vi "Main.vi"(11 "Module Admin":refnum<class "Delacor_lib_QMH_Module Admin.lvclass">) -> ()   [LabVIEW 2019, in "Panther Dashboard.lvlib"]
doc: "Panther Dashboard For DQMH®\n\nDeveloped and maintained by:\nPantherLAB\n\nMain Contributor- Developer:\n\n» Enrique Noé Arias\n\nBrainstorming & Code Reviews:\n\n» Matthias Baudot\n» Fabiola De La Cueva\n» Christopher Farmer\n» Cyril Gambini\n» Joerg Hampel\n» Olivier Jourdan\n» Cesar Muñoz\n» Darren Nattinger\n» Luis Orozco\n» Sam Taggart\n» Diego Torres"
uses:
  Panther Dashboard.lvlib
  <vilib>/Delacor/Delacor QMH/Libraries/Module Admin_class/Delacor_lib_QMH_Module Admin.lvclass
  Module Data--cluster.ctl
  Maps List and refs--cluster.ctl
  <vilib>/National Instruments/Tree Map/Tree Map Data.ctl
  DQMH Modules Info--cluster.ctl
  Module type--enum.ctl
  Project References--cluster.ctl
  Selection Type--enum.ctl
  References Updated Argument--cluster.ctl
  Launch DQMH Scripting Tools Argument--cluster.ctl
  DQMH Tools Menu--enum.ctl
  <vilib>/Delacor/Delacor QMH/Libraries/Message Queue_class/Delacor_lib_QMH_Message Queue.lvclass/Delacor_lib_QMH_Message Queue.ctl
  Expand Results Argument--cluster.ctl
  Execute Default Event Request Argument--cluster.ctl
  Tree DQMH Selection Argument--cluster.ctl
  Scan DQMH Modules Argument--cluster.ctl
  Stop Argument--cluster.ctl
  Generate Project Documentation Argument--cluster.ctl
  Set App Theme Argument--cluster.ctl
  Show About Argument--cluster.ctl
  Update Module ID Argument--cluster.ctl
  Save Library Description Argument--cluster.ctl
  Save VI Description Argument--cluster.ctl
  Open Documentation Argument--cluster.ctl
  Save Project Documentation Argument--cluster.ctl
  <vilib>/Delacor/Delacor QMH/Libraries/Module Admin_class/Delacor_lib_QMH_Module Admin.lvclass/Delacor_lib_QMH_Module Admin.ctl
  <vilib>/Delacor/Delacor QMH/Libraries/Message Queue_class/Delacor_lib_QMH_Enqueue Message (Single).vi
  <vilib>/Delacor/Delacor QMH/Libraries/Module Admin_class/Delacor_lib_QMH_Get External Launch.vi
  Panther Dashboard--global.vi
  <vilib>/National Instruments/Tree Map/API/List Roots.vi
  <vilib>/National Instruments/Tree Map/Utility/Into Tree Control Items.vi
  <vilib>/Platform/browser.llb/Open URL in Default Browser (path).vi
  <vilib>/Utility/error.llb/Error Cluster From Error Code.vi
  <vilib>/ErrorRing/Error Ring.xnode
  <vilib>/Delacor/Delacor QMH/Libraries/Message Queue_class/Delacor_lib_QMH_Message Queue.lvclass
  <vilib>/National Instruments/Tree Map/Tree Map.lvlib
  <vilib>/Delacor/Delacor QMH/Libraries/Scripting API/DQMH_Scripting API.lvlib
  ContextHelp/ContextHelp.lvlib
panel:
  out "error out":errorcluster
  in  "Context Help Panther":bool caption="Doc Editor"
  in  "Add Event":bool
  in  "Remove Event":bool caption="Remove"
  in  "Convert Event":bool caption="Convert"
  in  "Rename Event":bool caption="Rename"
  in  "Add New Module":bool caption="Add"
  in  "Rename Module":bool caption="Rename"
  in  "Validate Module":bool caption="Validate"
  in  "Create Module Template":bool caption="Template"
  in  "Add Unit Test Module":bool caption="Unit Test"
  in  "Create RT Tester Module":bool caption="RT Tester"
  in  "Open Antidoc Output":bool caption="Open"
  in  "Generate Antidoc":bool caption="Antidoc"
  in  "About Panther":bool caption="About"
  in  "Theme Panther":bool caption="Theme"
  in  "Projects":string(combo)
  in  "Targets":string(combo)
  in  "Search":bool caption="Scan Project"
  in  "Expand Results":bool
  in  "Include Dependencies":bool
  in  "Module ID":i32=-1 min=-1 max=1000 step=1 format="Module ID %d"
  in  "Modules Tree":string(tree) caption="Tree 2"
  out "antidoc":bool
  out "Panther Indicator":bool
  out "Process Indicator":bool
  out "Event Indicator":bool
  out "Status":string
  out "Progress":u16(slide) scale=-1.0..4.0
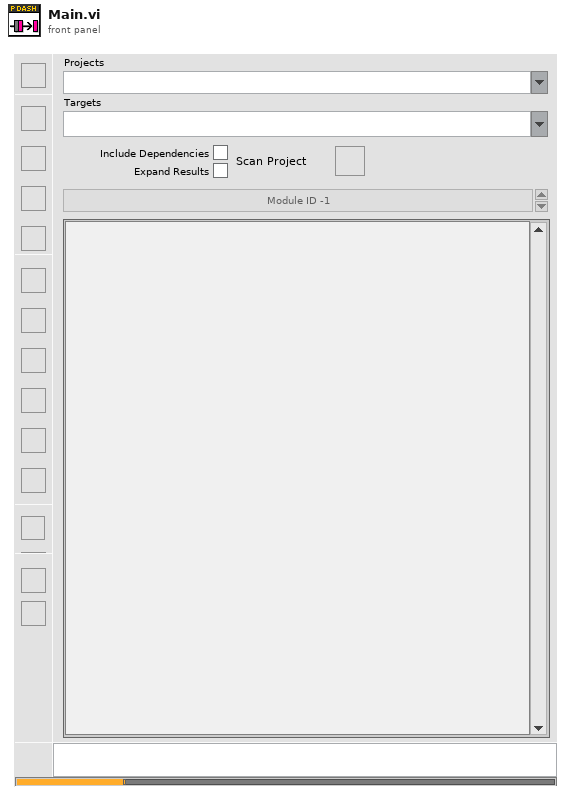
[diagram p1: front panel]
types:
  T1 = typedef "Panther Dashboard.lvlib/Broadcast Events--cluster.ctl" = cluster{"Module Did Init":refnum<user-event>, "Status Updated":refnum<user-event>, "Error Reported":refnum<user-event>, "Module Did Stop":refnum<user-event>, "Update Module Execution Status":refnum<user-event>, "References Updated":refnum<user-event>, "Projects Updated":refnum<user-event>, "Targets Updated":refnum<user-event>, "Progress updated":refnum<user-event>, "Scale Updated":refnum<user-event>, "Connector Pane Updated":refnum<user-event>, "Documentation Updated":refnum<user-event>, "Module Type Updated":refnum<user-event>, "Theme Updated":refnum<user-event>, "Project Description Updated":refnum<user-event>}
  T2 = typedef "Panther Dashboard.lvlib/Request Events--cluster.ctl" = cluster{"Stop Module":refnum<user-event>, "Show Panel":refnum<user-event>, "Hide Panel":refnum<user-event>, "Get Module Execution Status":refnum<user-event>, "Show Diagram":refnum<user-event>, "Scan DQMH Modules":refnum<user-event>, "Tree DQMH Selection":refnum<user-event>, "Open Module API Tester":refnum<user-event>, "Execute Default Event Request":refnum<user-event>, "Expand Results":refnum<user-event>, "Launch DQMH Scripting Tools":refnum<user-event>, "Generate Project Documentation":refnum<user-event>, "Set App Theme":refnum<user-event>, "Show About":refnum<user-event>, "Update Module ID":refnum<user-event>, "Save Library Description":refnum<user-event>, "Save VI Description":refnum<user-event>, "Open Documentation":refnum<user-event>, "Save Project Documentation":refnum<user-event>, "Register controls Mouse Enter":refnum<user-event>}
  T3 = typedef "ContextHelp.lvlib/Broadcast Events--cluster.ctl" = cluster{"Module Did Init":refnum<user-event>, "Status Updated":refnum<user-event>, "Error Reported":refnum<user-event>, "Module Did Stop":refnum<user-event>, "Update Module Execution Status":refnum<user-event>}
  T4 = typedef "Panther Dashboard.lvlib/Selection Type--enum.ctl" = enum16{"Broadcast", "Request", "Module", "Public API"}
  T5 = typedef "Panther Dashboard.lvlib/Module Data--cluster.ctl" = cluster{"Maps":T6, "DQMH Scan Results":T8, "Current Selection":cluster{"VI Ref":refnum<vi>, "DQMH Lib Ref":refnum<vi>}, "Module type":T9, "Module ID":i32, "Theme":bool, "Broadcast?":bool}
  T6 = typedef "Panther Dashboard.lvlib/Maps List and refs--cluster.ctl" = cluster{"Tree Map":T7, "References Map":map{string, refnum<vi>}}
  T7 = typedef "Tree Map.lvlib/Tree Map Data.ctl" = map{string, cluster{"Child Paths Set":set{string}, "Name":string, "Data":string, "Attributes":map{string, string}}}
  T8 = typedef "Panther Dashboard.lvlib/DQMH Modules Info--cluster.ctl" = cluster{"All DQMH Modules Refs":refnum<vi>[], "All Modules Descriptions":string[], "All Modules type":T9[], "Project References":T10}
  T9 = typedef "Panther Dashboard.lvlib/Module type--enum.ctl" = enum16{"Module type: Singleton", "Module type: Cloneable"}
  T10 = typedef "Panther Dashboard.lvlib/Project References--cluster.ctl" = cluster{"Project Ref":refnum<vi>, "Project Name":string, "Target":refnum<vi>, "App Ref":refnum<vi>}
  T11 = typedef "Panther Dashboard.lvlib/References Updated Argument--cluster.ctl" = cluster{"Modules":refnum<vi>[], "Modules Types":T9[], "Application Instance":refnum<vi>}
  T12 = enum8{"Enabled", "Disabled", "Disabled and Grayed Out"}
  T13 = typedef "Panther Dashboard.lvlib/Launch DQMH Scripting Tools Argument--cluster.ctl" = cluster{"Scripting Tool":T14}
  T14 = typedef "Panther Dashboard.lvlib/DQMH Tools Menu--enum.ctl" = enum16{"Create New DQMH Event", "Remove DQMH Event", "Convert DQMH Event", "Rename DQMH Event", "Add New DQMH Module", "Create RT Tester", "Rename DQMH Module", "Validate DQMH Module", "Create DQMH Module Template", "New DQMH  Unit Test"}
  T15 = typedef "Panther Dashboard.lvlib/Expand Results Argument--cluster.ctl" = cluster{"Expand?":bool}
  T16 = typedef "Panther Dashboard.lvlib/Execute Default Event Request Argument--cluster.ctl" = cluster{"Event Name":string}
  T17 = typedef "Panther Dashboard.lvlib/Tree DQMH Selection Argument--cluster.ctl" = cluster{"Tree DQMH Sel":string}
  T18 = typedef "Panther Dashboard.lvlib/Scan DQMH Modules Argument--cluster.ctl" = cluster{"Include Dependencies":bool, "Project":string, "Target":string}
  T19 = enum32{"invalid lock state", "Not Locked", "Locked (No Password)", "Password-protected"}
  T20 = typedef "Panther Dashboard.lvlib/Stop Argument--cluster.ctl" = cluster{"Origin":string, "Exit via Stop Module Req?":bool, "Wait for Module to stop?":bool}
  T21 = typedef "Panther Dashboard.lvlib/Generate Project Documentation Argument--cluster.ctl" = cluster{"Boolean":bool}
  T22 = typedef "Panther Dashboard.lvlib/Set App Theme Argument--cluster.ctl" = cluster{"Theme":bool}
  T23 = typedef "Panther Dashboard.lvlib/Show About Argument--cluster.ctl" = cluster{"Boolean":bool}
  T24 = typedef "Panther Dashboard.lvlib/Update Module ID Argument--cluster.ctl" = cluster{"New ID":i32}
  T25 = typedef "Panther Dashboard.lvlib/Save Library Description Argument--cluster.ctl" = cluster{"Library Description":string}
  T26 = typedef "Panther Dashboard.lvlib/Save VI Description Argument--cluster.ctl" = cluster{"VI Description":string}
  T27 = typedef "Panther Dashboard.lvlib/Open Documentation Argument--cluster.ctl" = cluster{"Boolean":bool}
  T28 = typedef "Panther Dashboard.lvlib/Save Project Documentation Argument--cluster.ctl" = cluster{"Project Description":string}
  T29 = cluster{"Left Cell String":string, "Child Text":string[], "Child Tag":string, "Item Indent":i32, "Child Only?":bool, "Glyph Index":i32}[]
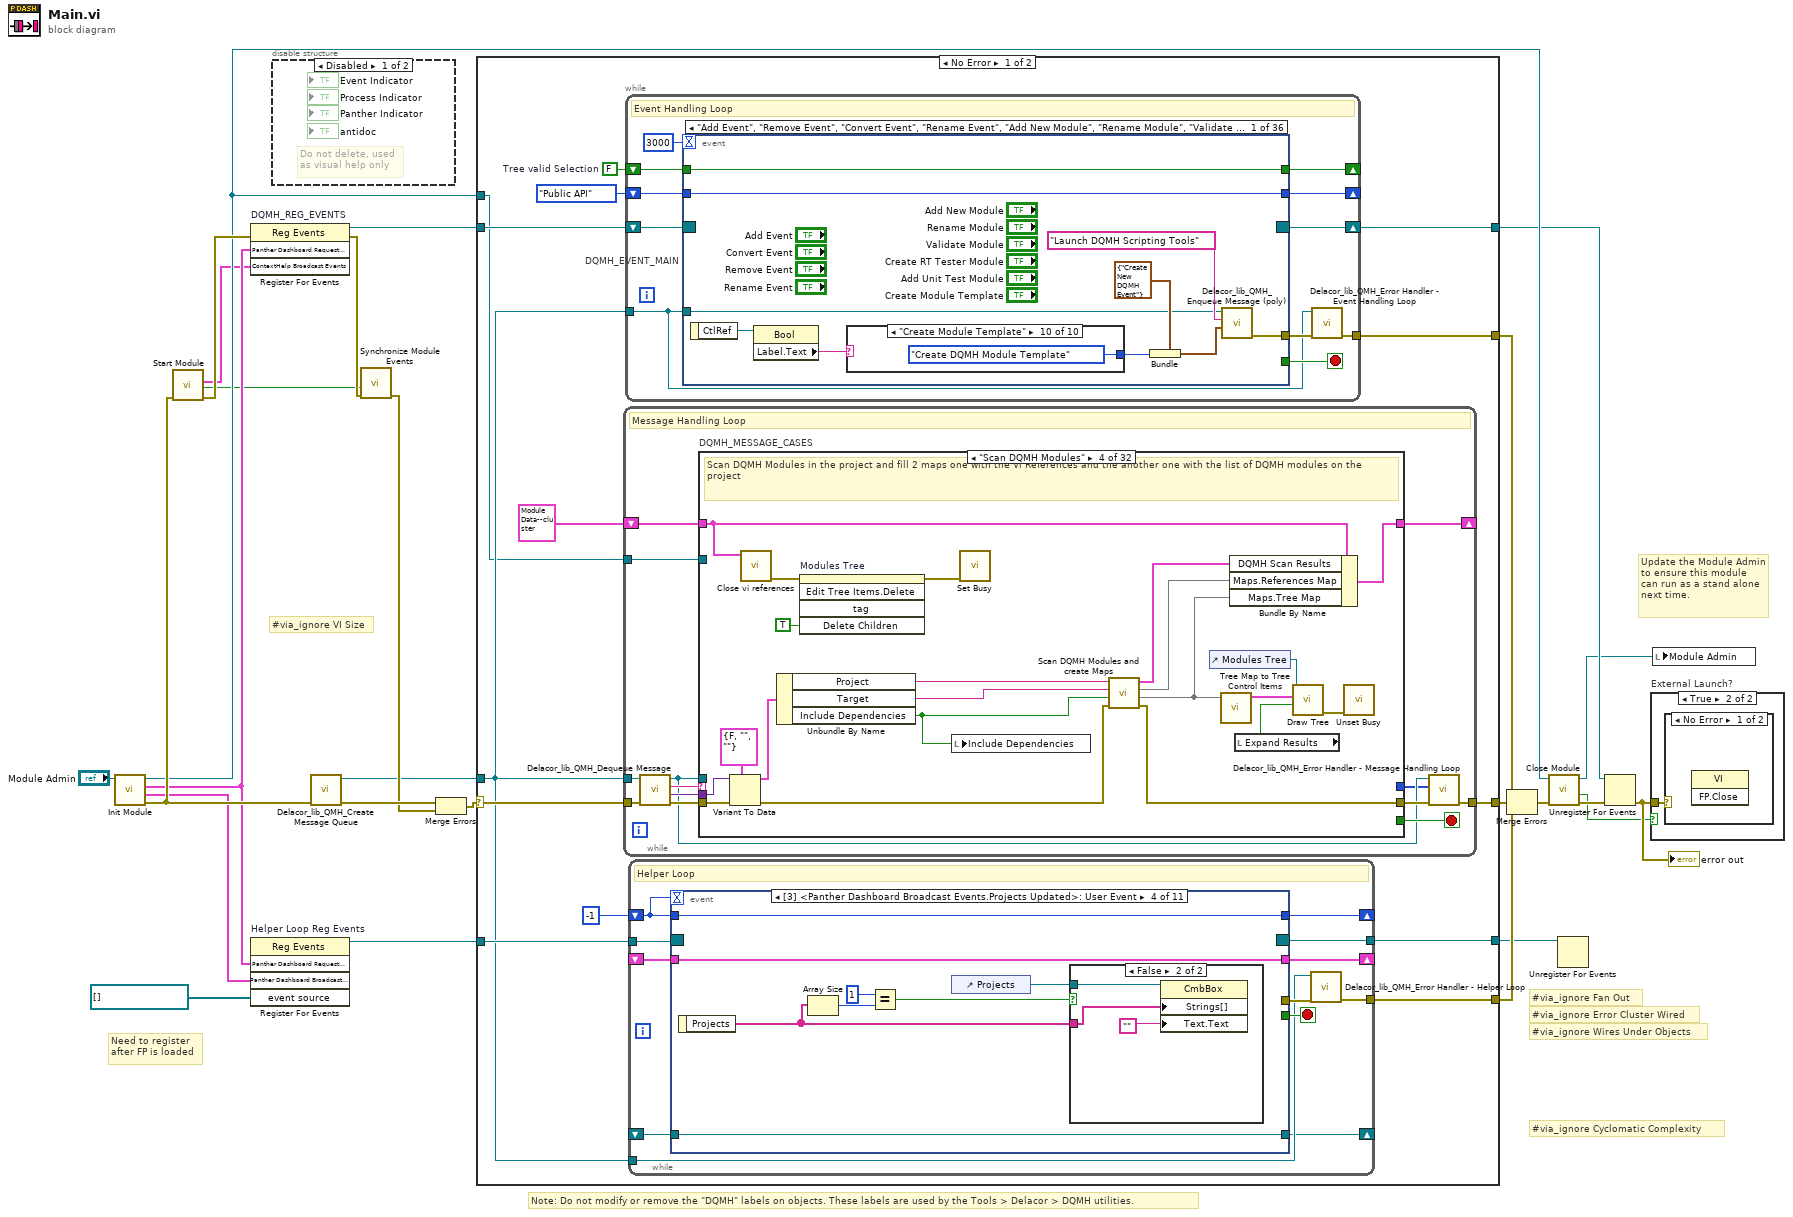
[diagram p0: block diagram]
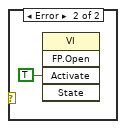
[diagram p4: hidden frame]
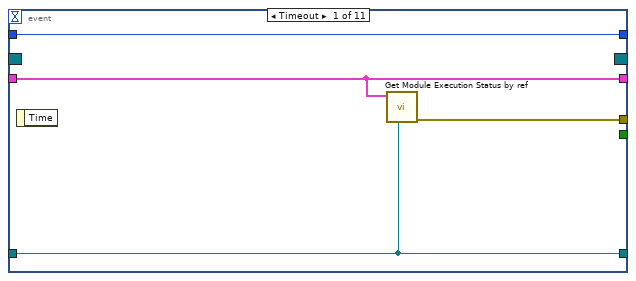
[diagram p5: hidden frame]
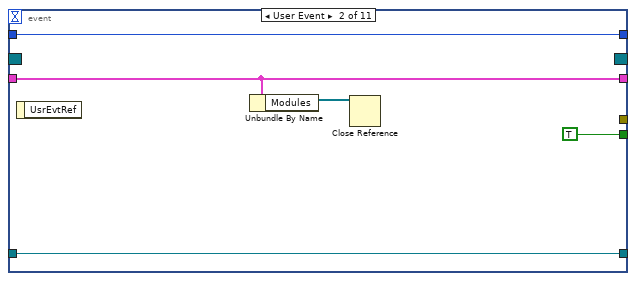
[diagram p6: hidden frame]
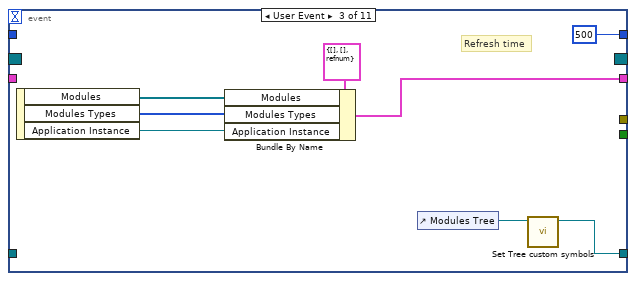
[diagram p7: hidden frame]
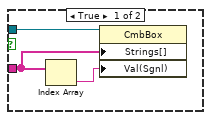
[diagram p8: hidden frame]
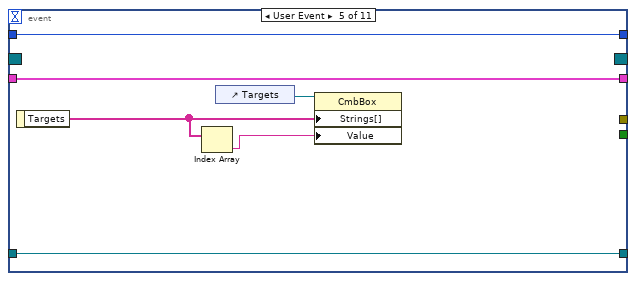
[diagram p9: hidden frame]
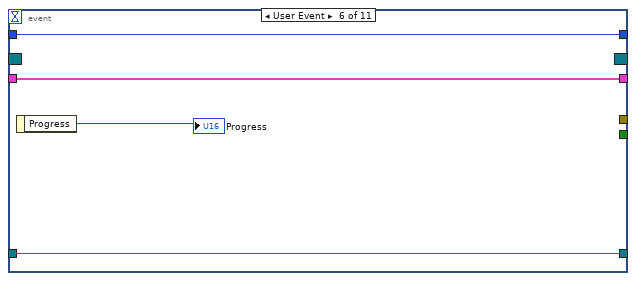
[diagram p10: hidden frame]
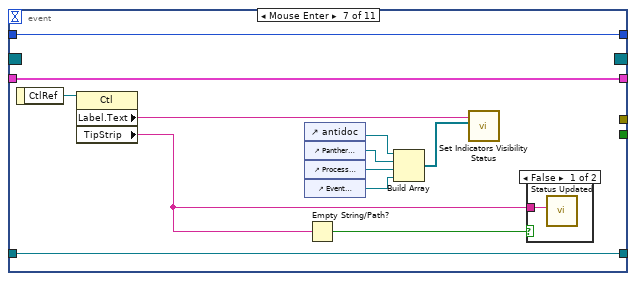
[diagram p11: hidden frame]
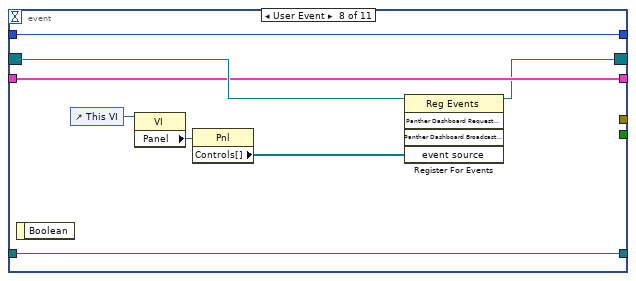
[diagram p13: hidden frame]
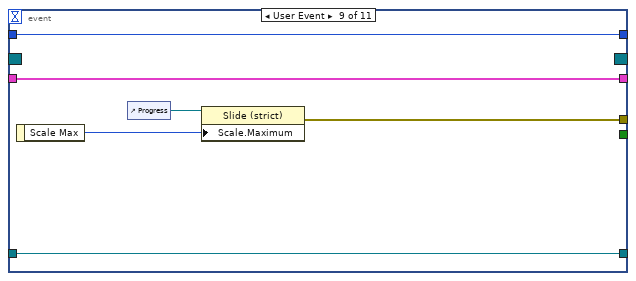
[diagram p14: hidden frame]
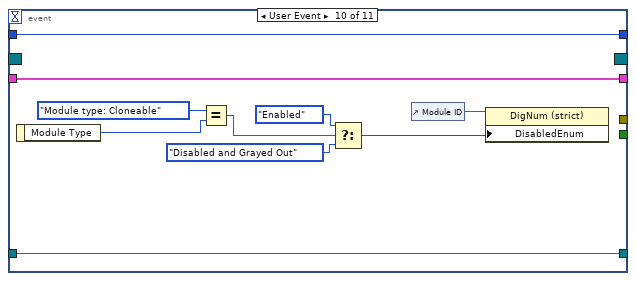
[diagram p15: hidden frame]
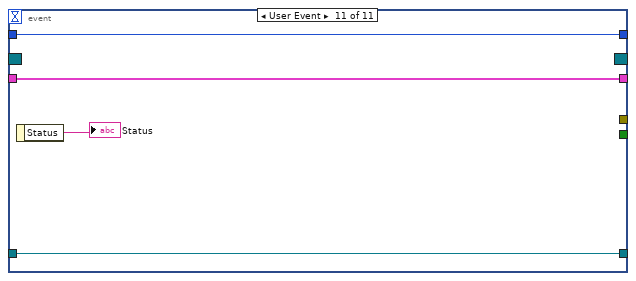
[diagram p16: hidden frame]
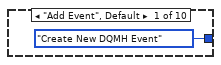
[diagram p17: hidden frame]
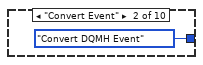
[diagram p18: hidden frame]
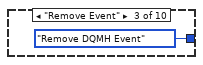
[diagram p19: hidden frame]
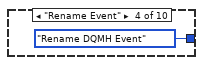
[diagram p20: hidden frame]
diagram:
  # "Need to register\nafter FP is loaded"
  # "#via_ignore VI Size"
  # "#via_ignore Fan Out"
  # "#via_ignore Cyclomatic Complexity"
  # "#via_ignore Wires Under Objects"
  # "#via_ignore Error Cluster Wired"
  # "Note: Do not modify or remove the \"DQMH\" labels on objects. These labels are used by the Tools > Delacor > DQMH utilities."
  # "Update the Module Admin to ensure this module can run as a stand alone next time."
  n1 = call "Init Module.vi"("Singleton Module Admin in"="Module Admin") -> ("error out"=w15:errorcluster, "Panther Dashboard Broadcast Events"=w4:T1, "Panther Dashboard Request Events"=w5:T2, "Singleton Module Admin out"=w14:refnum<class "Delacor_lib_QMH_Module Admin.lvclass">)  [unwired: 7 in]
  n2 = call "Start Module.vi"("error in"=w15) -> ("error out"=w17:errorcluster, "Wait for Event Sync?"=w3:bool, "ContextHelp Broadcast Events"=w2:T3)  [unwired: 7 in, 1 out]
  n3 = register-events "DQMH_REG_EVENTS"(error in=w17, w5, w2) -> (reference out=w12:refnum<event-registration>, error out=w18:errorcluster)  [unwired: 1 in]
  n4 = register-events "Helper Loop Reg Events"(w5, w4, refnum<vi>[] [] ("event source")) -> (reference out=w7:refnum<event-registration>)  [unwired: 2 in, 1 out]
  n5 = disable-structure shown="Disabled" {
    frame Disabled {
      # "Do not delete, used\nas visual help only"
    }
    frame Enabled {
    }
  }
  n6 = call <vilib>:"Delacor_lib_QMH_Create Message Queue.vi"("error in"=w15) -> ("error out"=w21:errorcluster, "Message Queue"=w11:refnum<class "Delacor_lib_QMH_Message Queue.lvclass">)  [unwired: 9 in]
  n7 = call "Synchronize Module Events.vi"("error in"=w18, "Wait for Event Sync?"=w3) -> ("error out"=w16:errorcluster)  [unwired: 9 in]
  n8 = Merge Errors(w21, w16) -> (w20:errorcluster)
  n9 = case shown="No Error" w20 {
    selector: w20 -> [w38 w805]
    tunnel: [w40 w804] -> w26
    tunnel: [w36 w803] -> w13
    tunnel: w12 -> [w34 w803]
    tunnel: w11 -> [w30 w799]
    tunnel: [w39 _] -> w24
    tunnel: w14 -> [w27 w800]
    tunnel: w7 -> [w33 w798]
    tunnel: [w32 w798] -> w6
    tunnel: [w37 _] -> w19
    frame No Error {
      w29 = FALSE  # Tree valid Selection
      n10 = while {
        tunnel: w30 -> [w451]
        shift-right: [w455] -> _
        shift-left: T5 {"Maps"={"Tree Map"={}, "References Map"={}}, "DQMH Scan Results"={"All DQMH Modules Refs"=[], "All Modules Descriptions"=[], "All Modules type"=[], "Project References"={"Project Ref"=refnum, "Project Name"="", "Target"=refnum, "App Ref"=refnum}}, "Current Selection"={"VI Ref"=refnum, "DQMH Lib Ref"=refnum}, "Module type"=enum."Module type: Singleton", "Module ID"=0, "Theme"=FALSE, "Broadcast?"=FALSE} ("Data Cluster") -> [w456]
        tunnel: w38 -> [w459]
        tunnel: [w457] -> w40
        tunnel: w27 -> [w449]
        stop <- w454 stop-if-true
        # "Message Handling Loop"
        n11 = call-dynamic "Delacor_lib_QMH_Dequeue Message.vi"("error in"=w459, "Message Queue in"=w451) -> ("error out"=w458:errorcluster, "Message Data"=w452:variant, "Message"=w453:string, "Message Queue out"=w450:refnum<class "Delacor_lib_QMH_Message Queue.lvclass">)  [unwired: 6 in]
        n12 = case "DQMH_MESSAGE_CASES" shown="\"Scan DQMH Modules\"" w453 {
          selector: w453 -> [_ w484 _ _ _ _ _ _ _ _ _ _ _ _ _ _ _ _ _ _ _ _ _ _ _ _ _ _ _ _ _ w784]
          tunnel: w450 -> [_ _ _ _ _ _ _ _ _ _ _ _ _ _ _ _ _ _ _ _ _ _ _ _ _ _ _ _ _ w753 w776 _]
          tunnel: w458 -> [w481 w489 w491 w512 w519 w526 w533 w548 w557 w562 w568 w582 w595 w617 w623 w630 w637 w642 w655 w664 w675 w684 w692 w702 w718 w734 w745 w748 w750 w760 w782 w786]
          tunnel: [w475 w487 w491 w511 w518 w526 w533 w547 w556 w563 w569 w580 w593 w618 w622 w629 w636 w641 w653 w662 w672 w680 w691 w700 w716 w733 w743 w747 w750 w756 w779 w787] -> w460
          tunnel: w456 -> [w472 w486 w490 w498 w516 w524 w532 w543 w555 w561 w567 w575 w592 w616 w621 w628 w635 w640 w644 w658 w671 w679 w690 w694 w711 w723 w739 w746 w749 w755 w768 w785]
          tunnel: [w471 w486 w490 w503 w516 w524 w532 w539 w555 w561 w567 w575 w592 w616 w621 w626 w635 w640 w644 w658 w666 w679 w686 w693 w709 w723 w739 w746 w749 w755 w768 w785] -> w455
          tunnel: [_ _ _ _ _ _ _ _ _ _ _ _ _ _ _ _ _ _ _ _ _ _ _ _ _ _ _ _ _ _ w775 _] -> w454
          tunnel: w452 -> [_ w485 _ w506 _ _ _ w546 _ _ _ w578 _ _ _ w627 w634 _ w652 w660 w670 w678 w689 w698 w714 w732 w742 _ _ w754 w774 _]
          tunnel: w449 -> [w473 _ _ _ _ _ _ _ _ _ _ _ _ _ _ _ _ _ _ _ _ _ _ _ _ _ _ _ _ w752 w769 _]
          tunnel: [_ _ _ _ _ _ _ _ _ _ _ _ i32[] [5000, 1026, 43] ("specific error code to clear (0: all)") _ _ _ _ _ _ _ _ _ _ _ _ _ _ _ _ _ _ _] -> w448
          frame "Initialize" {
            w462 = "Panther Dashboard for DQMH" ("format string")
            # "Initialize - Any operation that needs to be done before the module can receive messages. Synchronize Caller Events.vi will inform Start Module.vi that the module has launched and is ready to receive messages. Module Did Init.vi will broadcast that the module initialized."
            n13 = call "Synchronize Caller Events.vi"("error in (no error)"=w481, "Singleton Module Admin in"=w473) -> ("error out"=w480:errorcluster)  [unwired: 8 in, 1 out]
            n14 = property on="Modules Tree" class="Tree (strict)"("Allow Item Drag"=TRUE ("Drag/Drop:Allow Dragging"), "SelColor"=u32 8355711) -> ()  [unwired: 2 in, 2 out]
            n15 = call "Module Name--constant.vi"() -> ("Module Name"=w469:string)  [unwired: 11 in]
            n16 = call "Module Did Init.vi"("error in (no error)"=w480, "Initialized?"=TRUE, "Origin"=w469) -> ("error out"=w479:errorcluster)  [unwired: 8 in]
            n17 = control-ref of="Projects"() -> (w465:refnum<vi>)
            n18 = call "Scan For App Projects.vi"("error in"=w479, "Init?"=TRUE, "Projects Ref"=w465) -> ("error out"=w478:errorcluster)  [unwired: 8 in]
            n19 = call "Read Theme from Config.vi"("error in"=w478) -> ("error out"=w477:errorcluster, "Theme"=w461:bool)  [unwired: 9 in]
            n20 = local write "Theme Panther"(w461) -> ()
            n21 = call "Set App Theme.vi"("error in"=w477, "Theme"=w461) -> ("error out"=w476:errorcluster)  [unwired: 9 in]
            n22 = control-ref of="This VI"() -> (w463:refnum<vi>)
            n23 = Bundle By Name(cluster=w472, "Module ID"=-1) -> (w471:T5)
            n24 = call "Status Updated.vi"("Status"=w462) -> ()  [unwired: 10 in, 1 out]
            n25 = call "Set Panel Initial State.vi"("Title"=w462, "Main Vi Ref"=w463) -> ("error out"=w474:errorcluster)  [unwired: 9 in]
            n26 = Merge Errors(w474, w476) -> (w475:errorcluster)
          }
          frame "Refresh Targets" {
            # "When the User selects a Project triggers this task to scan all the targets available"
            n27 = Variant To Data(error in=w489, type=w484, Variant=w485) -> (data=w483:string, error out=w488:errorcluster)
            n28 = call "Get all Targets.vi"("error in"=w488, "Project Selection"=w483) -> ("error out"=w487:errorcluster, "Targets"=w482:string[])  [unwired: 8 in]
            n29 = call "Targets Updated.vi"("Targets"=w482) -> ()  [unwired: 10 in, 1 out]
          }
          frame "---Module Specific---" {
            # "Separator -- The following cases handle messages specific to this Module."
          }
          frame "Scan DQMH Modules" {
            # "Scan DQMH Modules in the project and fill 2 maps one with the Vi References and the another one with the list of DQMH modules on the project"
            n30 = Variant To Data(error in=w512, type=T18 {"Include Dependencies"=FALSE, "Project"="", "Target"=""} ("Scan DQMH Modules Argument"), Variant=w506) -> (data=w504:T18, error out=w509:errorcluster)
            n31 = call "Close vi references.vi"("Data Cluster"=w498) -> ("error out"=w508:errorcluster)  [unwired: 10 in]
            n32 = Unbundle By Name(w504) -> ("Project"=w494:string, "Target"=w496:string, "Include Dependencies"=w497:bool)
            n33 = invoke on="Modules Tree" class="Tree (strict)" method="Edit Tree Items.Delete"(error in=w508, "Delete Children"=TRUE ("Delete Children?")) -> (error out=w507:errorcluster)  [unwired: 3 in, 4 out]
            n34 = local write "Include Dependencies"(w497) -> ()
            n35 = call <vilib>:"Set Busy.vi"("error in (no error)"=w507) -> ()  [unwired: 9 in, 2 out]
            n36 = call "Scan DQMH Modules and create Maps.vi"("error in"=w509, "Include Dependencies"=w497, "Target Selection"=w496, "Project"=w494) -> ("error out"=w511:errorcluster, "Tree Map out"=w495:T7, "map ref out"=w499:map{string, refnum<vi>}, "DQMH Scan Results"=w502:T8)  [unwired: 4 in]
            n37 = control-ref of="Modules Tree"() -> (w500:refnum<vi>)
            n38 = call <vilib>:"Tree Map to Tree Control Items.vi"("Tree Map In"=w495) -> ("Tree Control Items"=w501:T29)  [unwired: 10 in]
            n39 = Bundle By Name(cluster=w498, "DQMH Scan Results"=w502, "Maps.References Map"=w499, "Maps.Tree Map"=w495) -> (w503:T5)
            n40 = local read "Expand Results"() -> (w492:bool)
            n41 = call "Draw Tree.vi"("Expanded Results?"=w492, "Tree Control Items"=w501, "TreeControl in"=w500) -> ("error out"=w510:errorcluster)  [unwired: 8 in]
            n42 = call <vilib>:"Unset Busy.vi"("error in (no error)"=w510) -> ()  [unwired: 10 in, 1 out]
          }
          frame "Drag VI" {
            # "This is the functionality alowing drag and drop the current selection to your code, you can build code using panther Dashboard."
            n43 = Unbundle By Name(w516) -> ("DQMH Scan Results.Project References.App Ref"=w515:refnum<vi>, "DQMH Scan Results.Project References.Target"=w514:refnum<vi>, "Current Selection.VI Ref"=w513:refnum<vi>)
            n44 = call "Drop Event into subVI.vi"("Current Selection.VI Ref"=w513, "Target"=w514, "App Ref"=w515) -> ("error out"=w517:errorcluster)  [unwired: 8 in]
            n45 = Merge Errors(w517, w519) -> (w518:errorcluster)
          }
          frame "Who is launching this module?" {
            w525 = 0  # Start Module.vi index
            # "Find all the VIS calling the Start Module.vi of the selected module library"
            n46 = Unbundle By Name(w524) -> ("Theme"=w523:bool, "DQMH Scan Results.Project References.App Ref"=w522:refnum<vi>, "DQMH Scan Results.Project References.Target"=w521:refnum<vi>, "Current Selection.DQMH Lib Ref"=w520:refnum<vi>)
            n47 = call "Find some Public API VI.vi"("Theme"=w523, "Public Api file index"=w525, "Library in"=w520, "Target"=w521, "App Ref"=w522) -> ()  [unwired: 7 in]
          }
          frame "Who is registered to this module's broadcasts?" {
            w531 = 2  # Obtain Broadcast Events for Registration.vi index
            # "Find all the VIS calling the Obtain broadcast events for registration of the selected module library"
            n48 = Unbundle By Name(w532) -> ("Theme"=w530:bool, "DQMH Scan Results.Project References.App Ref"=w529:refnum<vi>, "DQMH Scan Results.Project References.Target"=w528:refnum<vi>, "Current Selection.DQMH Lib Ref"=w527:refnum<vi>)
            n49 = call "Find some Public API VI.vi"("Theme"=w530, "Public Api file index"=w531, "Library in"=w527, "Target"=w528, "App Ref"=w529) -> ()  [unwired: 7 in]
          }
          frame "Tree DQMH Selection" {
            # "There is a new selection of the DQMH Tree list, need to search and update indicators acordanly."
            n50 = Unbundle By Name(w543) -> ("Maps.Tree Map"=w542:T7, "Maps.References Map"=w541:map{string, refnum<vi>}, "DQMH Scan Results"=w540:T8)
            n51 = Variant To Data(error in=w548, type=T17 {"Tree DQMH Sel"=""} ("Tree DQMH Selection Argument"), Variant=w546) -> (data=w544:T17, error out=w547:errorcluster)
            n52 = Unbundle By Name(w544) -> ("Tree DQMH Sel"=w536:string)
            n53 = call "Get List Information.vi"("List Selection"=w536, "DQMH Scan Info"=w540, "References Map"=w541, "Tree Map"=w542) -> ("Broadcast?"=w534:bool, "Vi out"=w537:refnum<vi>, "Module type"=w535:T9, "DQMH Lib"=w538:refnum<vi>)  [unwired: 4 in]
            n54 = Bundle By Name(cluster=w543, "Current Selection.DQMH Lib Ref"=w538, "Current Selection.VI Ref"=w537, "Module type"=w535, "Broadcast?"=w534) -> (w539:T5)
          }
          frame "Open Module API Tester" {
            # "If nothing selected use the first DQMH module"
            # "Open the API Tester from the current DQMH Module Selected"
            n55 = Unbundle By Name(w555) -> ("DQMH Scan Results.Project References.App Ref"=w554:refnum<vi>, "DQMH Scan Results.All DQMH Modules Refs"=w553:refnum<vi>[], "Current Selection.DQMH Lib Ref"=w549:refnum<vi>)
            n56 = Index Array(array=w553) -> (element=w551:refnum<vi>)  [unwired: 1 in]
            n57 = Not A Number/Path/Refnum?(number/path/refnum=w549) -> (NaN/Path/Refnum?=w552:bool)
            n58 = Select(t=w551, s=w552, f=w549) -> (s? t:f=w550:refnum<vi>)
            n59 = call "Open API Tester.vi"("error in"=w557, "DQMH Library Ref"=w550, "Application Instance"=w554) -> ("error out"=w556:errorcluster)  [unwired: 8 in]
          }
          frame "Find Module in project" {
            # "Find the selected module in project explorer"
            n60 = Unbundle By Name(w561) -> ("Current Selection.DQMH Lib Ref"=w560:refnum<vi>, "DQMH Scan Results.Project References.Project Ref"=w559:refnum<vi>, "DQMH Scan Results.All DQMH Modules Refs"=w558:refnum<vi>[])
            n61 = call "Find Library in Project.vi"("error in (no error)"=w562, "DQMH Modules Refs"=w558, "Project Ref"=w559, "DQMH Lib Ref"=w560) -> ("error out"=w563:errorcluster)  [unwired: 7 in]
          }
          frame "Locate Event on Main" {
            # "Find the selected event vi on the owing DQMH Module, if it is a reques we highlight its frame, if it is a broadcast we highlight where the broadcast is being triggered"
            n62 = Unbundle By Name(w567) -> ("DQMH Scan Results.Project References.App Ref"=w565:refnum<vi>, "Current Selection.VI Ref"=w566:refnum<vi>, "Broadcast?"=w564:bool)
            n63 = call "Find Event Frame.vi"("error in"=w568, "Broadcast?"=w564, "VI in"=w566, "Application Instance"=w565) -> ("error out"=w569:errorcluster)  [unwired: 7 in]
          }
          frame "Execute Default Event Request" {
            # "Execute Default Event"
            n64 = Variant To Data(error in=w582, type=T16 {"Event Name"=""} ("Execute Default Event Request Argument"), Variant=w578) -> (data=w576:T16, error out=w581:errorcluster)
            n65 = Unbundle By Name(w575) -> ("DQMH Scan Results.Project References.App Ref"=w574:refnum<vi>, "Current Selection.DQMH Lib Ref"=w573:refnum<vi>, "Module ID"=w571:i32, "Module type"=w570:T9)
            n66 = Unbundle By Name(w576) -> ("Event Name"=w572:string)
            n67 = call "Execute Default event.vi"("Module type"=w570, "Module ID"=w571, "Event"=w572, "DQMH Library Ref"=w573, "application Instance"=w574) -> ("error out"=w579:errorcluster)  [unwired: 6 in]
            n68 = Merge Errors(w581, w579) -> (w580:errorcluster)
          }
          frame "Search for Event Callers / listeners" {
            # "1026-Invalid Ref\n43- Operation\n canceled by user\n5000- something\nrandom happening\non DQMH Scripting\nAPI"
            # "Search for this event callers"
            n69 = Unbundle By Name(w592) -> ("DQMH Scan Results.Project References.Project Ref"=w586:refnum<vi>, "Current Selection.VI Ref"=w591:refnum<vi>, "Theme"=w583:bool, "Broadcast?"=w584:bool)
            n70 = Select(t="Searching code registered to broadcast selection" ("Status"), s=w584, f="Searching for Event Callers" ("Status")) -> (s? t:f=w587:string)
            n71 = call "Status Updated.vi"("error in (no error)"=w595, "Status"=w587) -> ("error out"=w594:errorcluster)  [unwired: 9 in]
            n72 = case shown="False" w584 {
              tunnel: w594 -> [w600 w607]
              tunnel: [w599 w606] -> w593
              tunnel: w591 -> [w598 w603]
              tunnel: [w597 w605] -> w590
              tunnel: w586 -> [w596 w604]
              frame False {
                # "Requests"
                n73 = call <vilib>:"Get Callers of Request VI in Project.vi"("error in"=w600, "Request VI"=w598, "Project"=w596) -> ("error out"=w599:errorcluster, "Request VI Callers"=w597:refnum<vi>[])  [unwired: 7 in]
              }
              frame True {
                # "Broadcast"
                n74 = Two Button Dialog(message="This is an exhaustive task that can take up to minutes, do you wish to continue?") -> (T button?=w602:bool)  [unwired: 2 in]
                n75 = case shown="False" w602 {
                  tunnel: w607 -> [w608 w613]
                  tunnel: [w608 w612] -> w606
                  tunnel: [_ w611] -> w605
                  tunnel: w604 -> [_ w610]
                  tunnel: w603 -> [_ w609]
                  frame False {
                  }
                  frame True {
                    n76 = call <vilib>:"Get VIs Registered for Broadcast in Project.vi"("error in"=w613, "Broadcast VI"=w609, "Project"=w610) -> ("error out"=w612:errorcluster, "VIs Registered for Broadcast"=w611:refnum<vi>[])  [unwired: 7 in]
                  }
                }
              }
            }
            n77 = call <vilib>:"Set Busy.vi"("error in (no error)"=w594) -> ()  [unwired: 9 in, 2 out]
            n78 = call <vilib>:"Unset Busy.vi"("error in (no error)"=w593) -> ()  [unwired: 10 in, 1 out]
            n79 = call "Start Call to results window.vi"("Find Broadcast?"=w584, "Request VI Callers"=w590, "Event"=w591, "Theme"=w583) -> ()  [unwired: 8 in]
          }
          frame "Open VI on Disk" {
            # "Open current event selection on the file system"
            n80 = Unbundle By Name(w616) -> ("Current Selection.VI Ref"=w615:refnum<vi>)
            n81 = property class="VI"(reference=w615) -> ("Path"=w614:path)  [unwired: 1 in, 2 out]
            n82 = call "Open File on Disk.vi"("error in"=w617, "file or directory path"=w614) -> ("error out"=w618:errorcluster)  [unwired: 9 in]
          }
          frame "Open File Library on Disk" {
            # "Open current Module Library selection on the file system"
            n83 = Unbundle By Name(w621) -> ("Current Selection.DQMH Lib Ref"=w620:refnum<vi>)
            n84 = property class="Library"(reference=w620) -> ("Path"=w619:path)  [unwired: 1 in, 2 out]
            n85 = call "Open File on Disk.vi"("error in"=w623, "file or directory path"=w619) -> ("error out"=w622:errorcluster)  [unwired: 9 in]
          }
          frame "Module ID Update" {
            # "Module ID Control has value change"
            n86 = Variant To Data(error in=w630, type=0 ("Module ID"), Variant=w627) -> (data=w625:i32, error out=w629:errorcluster)
            n87 = Bundle By Name(cluster=w628, "Module ID"=w625) -> (w626:T5)
          }
          frame "Expand or Close" {
            # "Expand or Close DQMH Tree control"
            n88 = Variant To Data(error in=w637, type=T15 {"Expand?"=FALSE} ("Expand or Close Argument"), Variant=w634) -> (data=w632:T15, error out=w636:errorcluster)
            n89 = Unbundle By Name(w632) -> ("Expand?"=w631:bool)
            n90 = invoke on="Modules Tree" class="Tree (strict)" method="Open/Close.Open/Close All"("Open"=w631) -> ()  [unwired: 3 in, 4 out]
          }
          frame "Open Project Folder" {
            n91 = Unbundle By Name(w640) -> ("DQMH Scan Results.Project References.Project Ref"=w639:refnum<vi>)
            n92 = property class="Project"(reference=w639) -> ("Path"=w638:path)  [unwired: 1 in, 2 out]
            n93 = call "Open File on Disk.vi"("error in"=w642, "file or directory path"=w638) -> ("error out"=w641:errorcluster)  [unwired: 9 in]
          }
          frame "Launch DQMH Scripting Tools" {
            # "Launch the DQMH Scripting Tools"
            n94 = Variant To Data(error in=w655, type=T13 {"Scripting Tool"=enum."Create New DQMH Event"} ("Launch DQMH Scripting Tools Argument"), Variant=w652) -> (data=w650:T13, error out=w654:errorcluster)
            n95 = Unbundle By Name(w650) -> ("Scripting Tool"=w645:T14)
            n96 = Unbundle By Name(w644) -> ("DQMH Scan Results.Project References.Project Name"=w648:string, "DQMH Scan Results.Project References.App Ref"=w649:refnum<vi>, "Current Selection.DQMH Lib Ref"=w643:refnum<vi>)
            n97 = Format Into String(format string="DQMH Tool: %s being executed ", w645) -> (resulting string=w647:string)  [unwired: 2 in, 1 out]
            n98 = call "Status Updated.vi"("Status"=w647) -> ()  [unwired: 10 in, 1 out]
            n99 = call "Launch DQMH Tools by menu.vi"("Project"=w648, "Application Instance"=w649, "error in"=w654, "Module Ref"=w643, "DQMH Tools"=w645) -> ("error out"=w653:errorcluster)  [unwired: 6 in]
          }
          frame "Generate Project Documentation" {
            n100 = Variant To Data(error in=w664, type=T21 {"Boolean"=FALSE} ("Generate Project Documentation Argument"), Variant=w660) -> (error out=w663:errorcluster)  [unwired: 1 out]
            n101 = Unbundle By Name(w658) -> ("DQMH Scan Results.Project References.Project Ref"=w657:refnum<vi>)
            n102 = property class="Project"(reference=w657) -> ("Path"=w656:path)  [unwired: 1 in, 2 out]
            n103 = call "Generate Documentation--dialog.vi"("Project Path"=w656) -> ("error out"=w661:errorcluster)  [unwired: 10 in]
            n104 = Merge Errors(w663, w661) -> (w662:errorcluster)
          }
          frame "Set App Theme" {
            # "Set Panther Dashboard Theme"
            n105 = Variant To Data(error in=w675, type=T22 {"Theme"=FALSE} ("Set App Theme Argument"), Variant=w670) -> (data=w668:T22, error out=w673:errorcluster)
            n106 = Unbundle By Name(w668) -> ("Theme"=w665:bool)
            n107 = control-ref of="This VI"() -> (w667:refnum<vi>)
            n108 = Bundle By Name(cluster=w671, "Theme"=w665) -> (w666:T5)
            n109 = call "Set Theme.vi"("Dark?"=w665, "VI in"=w667) -> ()  [unwired: 10 in]
            n110 = call "Theme Updated.vi"("Theme"=w665) -> ()  [unwired: 10 in, 1 out]
            n111 = call "Save Theme in config.vi"("error in"=w673, "Theme"=w665) -> ("error out"=w674:errorcluster)  [unwired: 9 in]
            n112 = call "Register controls Mouse Enter.vi"("error in"=w674) -> ("error out"=w672:errorcluster)  [unwired: 10 in]
          }
          frame "Show About" {
            # "Show About project"
            n113 = Variant To Data(error in=w684, type=T23 {"Boolean"=FALSE} ("Show About Argument"), Variant=w678) -> (error out=w681:errorcluster)  [unwired: 1 out]
            n114 = control-ref of="This VI"() -> (w676:refnum<vi>)
            n115 = call "Hide VI Panel.vi"("error in (no error)"=w681, "VI"=w676) -> ("error out"=w683:errorcluster)  [unwired: 9 in]
            n116 = call "About Panther Dashboard.vi"("error in"=w683) -> ("error out"=w682:errorcluster)  [unwired: 10 in]
            n117 = call "Open VI Panel.vi"("error in (no error)"=w682, "VI"=w676) -> ("error out"=w680:errorcluster)  [unwired: 9 in]
          }
          frame "Update Module ID" {
            # "Update the Current Module ID"
            n118 = Variant To Data(error in=w692, type=T24 {"New ID"=-1} ("Update Module ID Argument"), Variant=w689) -> (data=w687:T24, error out=w691:errorcluster)
            n119 = Unbundle By Name(w687) -> ("New ID"=w685:i32)
            n120 = Bundle By Name(cluster=w690, "Module ID"=w685) -> (w686:T5)
          }
          frame "Save Library Description" {
            # "Save Library Description"
            n121 = Variant To Data(error in=w702, type=T25 {"Library Description"=""} ("Save Library Description Argument"), Variant=w698) -> (data=w696:T25, error out=w701:errorcluster)
            n122 = Unbundle By Name(w696) -> ("Library Description"=w695:string)
            n123 = in-place {
              in-place-border: w695 -> [w706]
              in-place-border: [w708] -> w699
              n124 = in-place-cluster #1(w694) -> ("Current Selection.DQMH Lib Ref"=w707:refnum<vi>, "DQMH Scan Results"=w704:T8)
              n125 = call "Save Library Documentation.vi"("New Description"=w706, "DQMH Modules Info In"=w704, "Library in"=w707) -> ("error out"=w708:errorcluster, "DQMH Modules Info Out"=w705:T8, "Lib out"=w703:refnum<vi>)  [unwired: 6 in]
              n126 = in-place-cluster #1("Current Selection.DQMH Lib Ref"=w703, "DQMH Scan Results"=w705) -> (w693:T5)
            }
            n127 = Merge Errors(w701, w699) -> (w700:errorcluster)
          }
          frame "Save VI Description" {
            # "Save Event Description"
            n128 = Variant To Data(error in=w718, type=T26 {"VI Description"=""} ("Save VI Description Argument"), Variant=w714) -> (data=w712:T26, error out=w717:errorcluster)
            n129 = Unbundle By Name(w712) -> ("VI Description"=w710:string)
            n130 = in-place {
              in-place-border: w710 -> [w721]
              in-place-border: [w722] -> w715
              n131 = in-place-cluster #2(w711) -> ("Current Selection.VI Ref"=w720:refnum<vi>)
              n132 = call "Save Event Description.vi"("Event Description"=w721, "Event Ref in"=w720) -> ("error out"=w722:errorcluster, "Event Ref out"=w719:refnum<vi>)  [unwired: 8 in]
              n133 = in-place-cluster #2("Current Selection.VI Ref"=w719) -> (w709:T5)
            }
            n134 = Merge Errors(w717, w715) -> (w716:errorcluster)
          }
          frame "Open Documentation" {
            # "Open Antidoc Documentation"
            n135 = Variant To Data(error in=w734, type=T27 {"Boolean"=FALSE} ("Open Documentation Argument"), Variant=w732) -> (error out=w733:errorcluster)  [unwired: 1 out]
            n136 = Unbundle By Name(w723) -> ("DQMH Scan Results.Project References.Project Ref"=w730:refnum<vi>)
            n137 = property class="Project"(reference=w730) -> ("Path"=w729:path)  [unwired: 1 in, 2 out]
            n138 = Strip Path(path=w729) -> (stripped path=w728:path)  [unwired: 1 out]
            n139 = Build Path(base path=w728, name or relative path=path "Antidoc-Output/Project-Documentation.html") -> (appended path=w727:path)
            n140 = call <vilib>:"Check if File or Folder Exists.vi"("path"=w727) -> ("file or folder exists?"=w725:bool, "dup path"=w726:path)  [unwired: 8 in, 1 out]
            n141 = case shown="False" w725 {
              tunnel: w726 -> [_ w736]
              frame False {
                n142 = invoke on="Generate Antidoc" class="Bool" method="ObjHighlight"() -> ()  [unwired: 3 in, 3 out]
                n143 = call "Status Updated.vi"("Status"="No Antidoc Output has been found, please select a project and generate it first.") -> ()  [unwired: 10 in, 1 out]
              }
              frame True {
                n144 = call-poly <vilib>:"Open URL in Default Browser.vi"("path"=w736) -> ()  [unwired: 5 in, 2 out]
              }
            }
          }
          frame "Save Project Documentation" {
            n145 = Variant To Data(error in=w745, type=T28 {"Project Description"=""} ("Save Project Documentation Argument"), Variant=w742) -> (data=w740:T28, error out=w744:errorcluster)
            n146 = Unbundle By Name(w740) -> ("Project Description"=w737:string)
            n147 = Unbundle By Name(w739) -> ("DQMH Scan Results.Project References.Project Ref"=w738:refnum<vi>)
            n148 = property class="Project"(reference=w738, error in=w744, "Description"=w737) -> (error out=w743:errorcluster)  [unwired: 1 out]
          }
          frame "---Copy This Frame---" {
            # "Duplicate this frame when creating new messages.  Change this comment in the duplicated frame to describe this message."
            n149 = Merge Errors(w748) -> (w747:errorcluster)
          }
          frame "---Exit and Error Handling---" {
            # "Separator - The following cases handle errors and exit messages."
          }
          frame "Error" {
            # "Error - Check the error message data and respond accordingly. This message is sent by the \"Error Handler\" VIs at the end of each loop in this application."
            n150 = property on="Property Node" class="Module Admin"(reference=w752) -> ("Accessors:External Launch"=w751:bool)  [unwired: 1 in, 2 out]
            n151 = Variant To Data(error in=w760, type=errorcluster {"status"=FALSE, "code"=0, "source"=""} ("error constant"), Variant=w754) -> (data=w761:errorcluster, error out=w758:errorcluster)
            n152 = call "Error Reported.vi"("Error"=w761) -> ()  [unwired: 10 in, 1 out]
            n153 = case shown="True" w751 {
              tunnel: [w766 _] -> w757
              tunnel: w753 -> [w764 _]
              tunnel: w761 -> [w765 _]
              frame False {
                # "If the module is running standalone, then pop up an error dialog and call the \"Exit\" message."
                n154 = call <vilib>:"Simple Error Handler.vi"("error in (no error)"=w765) -> ()  [unwired: 4 in, 5 out]
                n155 = call-poly <vilib>:"Delacor_lib_QMH_Enqueue Message (poly).vi"("Priority Message? (F)"=TRUE, "Message"="Exit", "Message Queue in"=w764) -> ("error out"=w766:errorcluster)  [unwired: 7 in, 1 out]
              }
              frame True {
                # "If the module was launched externally, calling the Error Reported broadcast VI is the only action performed by the \"Error\" message. The module's caller can then process the error appropriately."
              }
            }
            n156 = Merge Errors(w758, w757) -> (w756:errorcluster)
            n157 = local write "error out"(w756) -> ()
          }
          frame "Exit" {
            w773 = 91  # 91: not all Exit messages will have an argument
            w775 = TRUE  # Stop the VI
            # "Release the message queue reference"
            # "Exit - Exit the application."
            n158 = Variant To Data(error in=w782, type=T20 {"Origin"="", "Exit via Stop Module Req?"=FALSE, "Wait for Module to stop?"=FALSE} ("Stop Argument"), Variant=w774) -> (data=w771:T20, error out=w778:errorcluster)
            n159 = call <vilib>:"Clear Errors.vi"("error in (no error)"=w778, "specific error code to clear (0: all)"=w773) -> ("error out"=w781:errorcluster)  [unwired: 4 in, 1 out]
            n160 = control-ref of="This VI"() -> (w770:refnum<vi>)
            n161 = invoke on="Modules Tree" class="Tree (strict)" method="Edit Tree Items.Delete"() -> ()  [unwired: 5 in, 5 out]
            n162 = call-dynamic "Delacor_lib_QMH_Release Message Queue.vi"("error in"=w781, "Message Queue"=w776) -> ("error out"=w780:errorcluster)  [unwired: 9 in]
            n163 = call "Handle Exit.vi"("Stop Argument"=w771, "Admin in"=w769, "VI reference"=w770) -> ("error out"=w777:errorcluster)  [unwired: 7 in, 1 out]
            n164 = call "Close vi references.vi"("Data Cluster"=w768) -> ()  [unwired: 10 in, 1 out]
            n165 = Merge Errors(w780, w777) -> (w779:errorcluster)
            n166 = call "Stop Module.vi"("Origin"="Panther Dahsboard Stopped") -> ()  [unwired: 10 in, 1 out]
          }
          frame Default {
            # "'Default' case only runs if there is a message that isn't defined in any of the other cases.  Output a programming error."
            n167 = call "Module Name--constant.vi"() -> ("Module Name"=w783:string)  [unwired: 11 in]
            n168 = xnode ("Error Ring")("parameter 0"=w784, "parameter 1"=w783) -> ("error out"=w788:errorcluster)
            n169 = Merge Errors(w786, w788) -> (w787:errorcluster)
          }
        }
        n170 = call-dynamic "Delacor_lib_QMH_Error Handler - Message Handling Loop.vi"("error in"=w460, "Ignore Errors (Runtime)"=w448, "Message Queue in"=w450) -> ("dup error in"=w457:errorcluster)  [unwired: 7 in, 1 out]
      }
      n171 = while {
        tunnel: w30 -> [w140]
        shift-right: [w142] -> w36
        shift-left: w34 -> [w143]
        tunnel: [w144] -> w39
        shift-right: [w138] -> _
        shift-left: w29 -> [w137]
        shift-right: [w136] -> _
        shift-left: Selection_Type--enum."Public API" ("Selection type") -> [w135]
        stop <- w141 stop-if-true
        # "Event Handling Loop"
        n172 = event "DQMH_EVENT_MAIN" shown="[0] \"Add Event\", \"Remove Event\", \"Convert Event\", \"Rename Event\", \"Add New Module\", \"Rename Module\", \"Validate Module\", \"Create Module Template\", \"Add Unit Test Module\", \"Create RT Tester Module\": Value Change" {
          selector: w143 -> [_ _ _ _ _ _ _ _ _ _ _ _ _ _ _ _ _ _ _ _ _ _ _ _ _ _ _ _ _ _ _ _ _ _ _ _]
          dyn-events: [_ _ _ _ _ _ _ _ _ _ _ _ _ _ _ _ _ _ _ _ _ _ _ _ _ _ _ _ _ _ _ _ _ _ _ _] -> w142
          timeout: 3000 -> [_ _ _ _ _ _ _ _ _ _ _ _ _ _ _ _ _ _ _ _ _ _ _ _ _ _ _ _ _ _ _ _ _ _ _ _]
          tunnel: [_ _ _ _ _ _ _ _ _ _ _ _ _ _ _ _ _ _ _ TRUE ("Discard?") _ _ _ _ _ _ _ _ _ _ _ _ _ _ _ _] -> w141
          tunnel: w140 -> [w146 _ _ w181 w186 w198 w203 w228 _ w237 _ w251 w261 _ _ w278 w287 _ _ w320 w329 _ w340 w348 w356 w364 w372 w380 w388 w396 w404 w412 w420 w428 w436 w444]
          tunnel: [w155 w169 w174 w182 w187 w199 w204 w229 w234 w240 w248 w254 w262 w266 _ w279 w288 _ _ w323 w331 w335 w343 w351 w359 w367 w375 w383 w391 w399 w407 w415 w423 w431 w439 w447] -> w145
          tunnel: [w154 w168 w173 w176 w184 w195 w201 w224 w230 w239 w247 w253 w256 w264 w268 w272 w285 w300 w311 w313 w326 w334 w342 w350 w358 w366 w374 w382 w390 w398 w406 w414 w422 w430 w438 w446] -> w138
          tunnel: w137 -> [w154 w168 w173 w176 w184 w195 w201 _ w230 w239 w247 w253 w256 w264 w268 w272 w285 w300 w311 w313 w326 w334 w342 w350 w358 w366 w374 w382 w390 w398 w406 w414 w422 w430 w438 w446]
          tunnel: [w153 w167 w172 w175 w183 w194 w200 w222 w232 w238 w246 w252 w255 w263 w267 w271 w284 w299 w310 w312 w325 w333 w341 w349 w357 w365 w373 w381 w389 w397 w405 w413 w421 w429 w437 w445] -> w136
          tunnel: w135 -> [w153 w167 w172 w175 _ w194 w200 _ w232 w238 w246 w252 w255 w263 w267 w271 w284 w299 w310 w312 w325 w333 w341 w349 w357 w365 w373 w381 w389 w397 w405 w413 w421 w429 w437 w445]
          event "Add Event", "Remove Event", "Convert Event", "Rename Event", "Add New Module", "Rename Module", "Validate Module", "Create Module Template", "Add Unit Test Module", "Create RT Tester Module": Value Change {
            n173 = event-data() -> ("CtlRef"=w151:refnum<vi>)  [unwired: 1 in]
            n174 = property class="Bool"(reference=w151) -> ("Label.Text"=w152:string)  [unwired: 1 in, 2 out]
            n175 = case shown="\"Create Module Template\"" w152 {
              tunnel: [DQMH_Tools_Menu--enum."Create New DQMH Event" ("DQMH Tools") DQMH_Tools_Menu--enum."Convert DQMH Event" ("DQMH Tools") DQMH_Tools_Menu--enum."Remove DQMH Event" ("DQMH Tools") DQMH_Tools_Menu--enum."Rename DQMH Event" ("DQMH Tools") DQMH_Tools_Menu--enum."Add New DQMH Module" ("DQMH Tools") DQMH_Tools_Menu--enum."Rename DQMH Module" ("DQMH Tools") DQMH_Tools_Menu--enum."Validate DQMH Module" ("DQMH Tools") DQMH_Tools_Menu--enum."Create RT Tester" ("DQMH Tools") DQMH_Tools_Menu--enum."New DQMH  Unit Test" ("DQMH Tools") DQMH_Tools_Menu--enum."Create DQMH Module Template" ("DQMH Tools")] -> w147
              frame "Add Event", Default {
              }
              frame "Convert Event" {
              }
              frame "Remove Event" {
              }
              frame "Rename Event" {
              }
              frame "Add New Module" {
              }
              frame "Rename Module" {
              }
              frame "Validate Module" {
              }
              frame "Create RT Tester Module" {
              }
              frame "Add Unit Test Module" {
              }
              frame "Create Module Template" {
              }
            }
            n176 = Bundle(cluster=T13 {"Scripting Tool"=enum."Create New DQMH Event"} ("Launch DQMH Scripting Tools Argument"), "Scripting Tool"=w147) -> (w150:T13)
            n177 = call-poly <vilib>:"Delacor_lib_QMH_Enqueue Message (poly).vi"("Message Data"=w150, "Message"="Launch DQMH Scripting Tools", "Message Queue in"=w146) -> ("error out"=w155:errorcluster)  [unwired: 7 in, 1 out]
          }
          event "Context Help Panther": Value Change {
            # "Open Documentation DQMH Module"
            n178 = event-data() -> ()  [unwired: 1 in, 1 out]
            n179 = case shown="True" "Context Help Panther" {
              tunnel: [w170 w171] -> w169
              frame False {
                n180 = call "Hide Panel.vi"() -> ("error out"=w170:errorcluster)  [unwired: 11 in]
              }
              frame True {
                n181 = call "Show Panel.vi"() -> ("error out"=w171:errorcluster)  [unwired: 11 in]
              }
            }
          }
          event User Event {
            # "We wait for the Context help module to init to request to refresh \npanther Dashboard Broadcasts, we need this module to be\nlistening Panther Dashboard broadcasts"
            n182 = event-data() -> ()  [unwired: 1 in, 1 out]
            n183 = call "Refresh Panther Dashboard Broadcasts.vi"() -> ("error out"=w174:errorcluster)  [unwired: 11 in]
          }
          event "Expand Results": Value Change {
            # "Expand or close Result tree"
            n184 = event-data() -> ()  [unwired: 1 in, 1 out]
            n185 = Bundle(cluster=T15 {"Expand?"=FALSE} ("Expand or Close Argument"), "Expand?"="Expand Results") -> (w178:T15)
            n186 = call-poly <vilib>:"Delacor_lib_QMH_Enqueue Message (poly).vi"("Message Data"=w178, "Message"="Expand or Close", "Message Queue in"=w181) -> ("error out"=w182:errorcluster)  [unwired: 7 in, 1 out]
          }
          event "Modules Tree": Double Click {
            # "User double click an element on the tree control, we check if it is an event to find its frame on the corresponding DQMH module, we also check if it is a broadcast to find where is being triggered"
            n187 = event-data() -> ("Tag"=w185:string)  [unwired: 1 in]
            n188 = call "Validate if event is selected.vi"("Tree Selection"=w185) -> ("Selection type"=w183:T4)  [unwired: 10 in]
            n189 = case shown="\"Module\"" w183 {
              tunnel: [w190 _ w193] -> w187
              tunnel: w186 -> [w189 _ w192]
              frame "Module" {
                # "Selection is a module"
                n190 = call-poly <vilib>:"Delacor_lib_QMH_Enqueue Message (poly).vi"("Message"="Find Module in project", "Message Queue in"=w189) -> ("error out"=w190:errorcluster)  [unwired: 8 in, 1 out]
              }
              frame "Public API" {
              }
              frame "Broadcast", "Request" {
                # "Selection is an Event vi?"
                n191 = call-poly <vilib>:"Delacor_lib_QMH_Enqueue Message (poly).vi"("Message"="Locate Event on Main", "Message Queue in"=w192) -> ("error out"=w193:errorcluster)  [unwired: 8 in, 1 out]
              }
            }
          }
          event "Modules Tree": Drag Starting? {
            # "Drag current selection to user destination"
            n192 = event-data() -> ()  [unwired: 1 in, 1 out]
            n193 = call-poly <vilib>:"Delacor_lib_QMH_Enqueue Message (poly).vi"("Message"="Drag VI", "Message Queue in"=w198) -> ("error out"=w199:errorcluster)  [unwired: 8 in, 1 out]
            n194 = event-data("Discard?"=TRUE) -> ()  [unwired: 1 in, 1 out]
          }
          event "Modules Tree": Shortcut Menu Selection (User) {
            # "User selects something from the Right Click Shortcut Menu"
            n195 = event-data() -> ("ItemTag"=w202:string)  [unwired: 1 in]
            n196 = case shown="\"Open File Library on Disk\", \"Open VI on Disk\", \"Who is launching this module?\"" w202 {
              selector: w202 -> [w207 _ w213 w216 w219]
              tunnel: w203 -> [w211 _ w214 w217 w220]
              tunnel: [w212 _ w215 w218 w221] -> w204
              frame "-Run: Hide Panel", "-Run: Show Diagram", "-Run: Show Panel", "-Run: Stop Module" {
                n197 = Match Pattern(string=w207, regular expression="-Run: ") -> (after substring=w206:string)  [unwired: 1 in, 3 out]
                n198 = Bundle(cluster=T16 {"Event Name"=""} ("Execute Default Event Request Argument"), "Event Name"=w206) -> (w209:T16)
                n199 = call-poly <vilib>:"Delacor_lib_QMH_Enqueue Message (poly).vi"("Message Data"=w209, "Message"="Execute Default Event Request", "Message Queue in"=w211) -> ("error out"=w212:errorcluster)  [unwired: 7 in, 1 out]
              }
              frame Default {
              }
              frame "Open File Library on Disk", "Open VI on Disk", "Who is launching this module?" {
                n200 = call-poly <vilib>:"Delacor_lib_QMH_Enqueue Message (poly).vi"("Message"=w213, "Message Queue in"=w214) -> ("error out"=w215:errorcluster)  [unwired: 8 in, 1 out]
              }
              frame "Who is registered to this module's broadcasts?" {
                n201 = call-poly <vilib>:"Delacor_lib_QMH_Enqueue Message (poly).vi"("Message"=w216, "Message Queue in"=w217) -> ("error out"=w218:errorcluster)  [unwired: 8 in, 1 out]
              }
              frame "Open Module API Tester", "Search for Event Callers / listeners" {
                n202 = call-poly <vilib>:"Delacor_lib_QMH_Enqueue Message (poly).vi"("Message"=w219, "Message Queue in"=w220) -> ("error out"=w221:errorcluster)  [unwired: 8 in, 1 out]
              }
            }
          }
          event "Modules Tree": Value Change {
            w224 = TRUE  # Tree valid Selection
            # "The user selected an item on the tree control"
            n203 = event-data() -> ()  [unwired: 1 in, 1 out]
            n204 = Bundle(cluster=T17 {"Tree DQMH Sel"=""} ("Tree DQMH Selection Argument"), "Tree DQMH Sel"="Modules Tree") -> (w225:T17)
            n205 = call "Validate if event is selected.vi"("Tree Selection"="Modules Tree") -> ("Selection type"=w222:T4)  [unwired: 10 in]
            n206 = call-poly <vilib>:"Delacor_lib_QMH_Enqueue Message (poly).vi"("Message Data"=w225, "Message"="Tree DQMH Selection", "Message Queue in"=w228) -> ("error out"=w229:errorcluster)  [unwired: 7 in, 1 out]
          }
          event "Modules Tree": Shortcut Menu Activation? {
            # "This is wher the shorcut menu is filled, only after the user select a module"
            n207 = event-data() -> ("MenuRef"=w233:refnum<k9>)  [unwired: 1 in]
            n208 = call "Create Tree Shortcut Menu.vi"("Selection type"=w232, "Menu in"=w233) -> ("error out"=w234:errorcluster)  [unwired: 9 in]
            n209 = Not(x=w230) -> (.not. x?=w231:bool)
            n210 = event-data("Discard?"=w231) -> ()  [unwired: 1 in, 1 out]
          }
          event "Projects": Value Change {
            n211 = event-data() -> ()  [unwired: 1 in, 1 out]
            n212 = call-poly <vilib>:"Delacor_lib_QMH_Enqueue Message (poly).vi"("Message Data"="Projects", "Message"="Refresh Targets", "Message Queue in"=w237) -> ("error out"=w240:errorcluster)  [unwired: 7 in, 1 out]
          }
          event "Projects": Shortcut Menu Activation? {
            n213 = event-data() -> ("MenuRef"=w245:refnum<k9>)  [unwired: 1 in]
            n214 = Delete Menu Items(9:w245) -> (0:w249:errorcluster, 3:w244:refnum<k9>)  [unwired: 3 in]
            n215 = Insert Menu Items(6:w249, 8:string[] ["Open Project Folder"] ("item names"), 9:w244) -> (0:w248:errorcluster)  [unwired: 3 in, 2 out]
            n216 = local read "Projects"() -> (w242:string)
            n217 = Empty String/Path?(string/path=w242) -> (empty?=w241:bool)
            n218 = event-data("Discard?"=w241) -> ()  [unwired: 1 in, 1 out]
          }
          event "Projects": Shortcut Menu Selection (User) {
            n219 = event-data() -> ("ItemTag"=w250:string)  [unwired: 1 in]
            n220 = call-poly <vilib>:"Delacor_lib_QMH_Enqueue Message (poly).vi"("Message"=w250, "Message Queue in"=w251) -> ("error out"=w254:errorcluster)  [unwired: 8 in, 1 out]
          }
          event User Event {
            # "Another Module called the \"Expand or Close\" API Method."
            n221 = event-data() -> ("Expand?"=w257:bool)  [unwired: 1 in]
            n222 = Bundle(cluster=T15 {"Expand?"=FALSE} ("Expand or Close Argument"), "Expand?"=w257) -> (w258:T15)
            n223 = call-poly <vilib>:"Delacor_lib_QMH_Enqueue Message (poly).vi"("Message Data"=w258, "Message"="Expand or Close", "Message Queue in"=w261) -> ("error out"=w262:errorcluster)  [unwired: 7 in, 1 out]
          }
          event User Event {
            # "Another Module called the \"Get Module Execution Status\" API Method."
            n224 = event-data() -> ()  [unwired: 1 in, 1 out]
            n225 = call "Update Module Execution Status.vi"("Running?"=TRUE) -> ("error out"=w266:errorcluster)  [unwired: 10 in]
          }
          event User Event {
            # "Hide the panel of this VI, and send a status updated message to let listeners know."
            # "Another Module called the \"Hide Panel\" API Method."
            n226 = event-data() -> ()  [unwired: 1 in, 1 out]
            n227 = control-ref of="This VI"() -> (w269:refnum<vi>)
            n228 = call "Hide VI Panel.vi"("VI"=w269) -> ()  [unwired: 10 in, 1 out]
          }
          event User Event {
            # "Another Module called the \"Scan DQMH Modules\" API Method."
            n229 = event-data() -> ("Include Dependencies"=w274:bool, "Project"=w273:string, "Target"=w270:string)  [unwired: 1 in]
            n230 = Bundle(cluster=T18 {"Include Dependencies"=FALSE, "Project"="", "Target"=""} ("Scan DQMH Modules Argument"), "Include Dependencies"=w274, "Project"=w273, "Target"=w270) -> (w275:T18)
            n231 = call-poly <vilib>:"Delacor_lib_QMH_Enqueue Message (poly).vi"("Message Data"=w275, "Message"="Scan DQMH Modules", "Message Queue in"=w278) -> ("error out"=w279:errorcluster)  [unwired: 7 in, 1 out]
          }
          event "Search": Value Change {
            # "#via_ignore Unwired Event Nodes"
            # "Another Module called the \"Scan DQMH Modules\" API Method."
            n232 = event-data() -> ()  [unwired: 1 in, 1 out]
            n233 = local read "Projects"() -> (w283:string)
            n234 = Empty String/Path?(string/path="Targets") -> (empty?=w281:bool)
            n235 = global write "Panther Dashboard--global.vi" "Target"("Targets") -> ()
            n236 = Empty String/Path?(string/path=w283) -> (empty?=w286:bool)
            n237 = Or(x=w286, y=w281) -> (x .or. y?=w282:bool)
            n238 = case shown="True" w282 {
              tunnel: [w296 _] -> w288
              tunnel: w287 -> [w295 _]
              tunnel: w283 -> [w290 _]
              tunnel: "Targets" -> [w289 _]
              frame False {
                n239 = Bundle(cluster=T18 {"Include Dependencies"=FALSE, "Project"="", "Target"=""} ("Scan DQMH Modules Argument"), "Include Dependencies"="Include Dependencies", "Project"=w290, "Target"=w289) -> (w292:T18)
                n240 = call-poly <vilib>:"Delacor_lib_QMH_Enqueue Message (poly).vi"("Message Data"=w292, "Message"="Scan DQMH Modules", "Message Queue in"=w295) -> ("error out"=w296:errorcluster)  [unwired: 7 in, 1 out]
              }
              frame True {
                n241 = invoke on="Projects" class="CmbBox" method="ObjHighlight"() -> (error out=w298:errorcluster)  [unwired: 3 in, 2 out]
                n242 = invoke on="Targets" class="CmbBox" method="ObjHighlight"(error in=w298) -> ()  [unwired: 2 in, 3 out]
                n243 = call "Status Updated.vi"("Status"="Scanning requires a project and an target please make the selection.\n") -> ()  [unwired: 10 in, 1 out]
              }
            }
          }
          event User Event {
            # "Another Module called the \"Show Diagram\" API Method. This event is used for debugging."
            n244 = event-data() -> ()  [unwired: 1 in, 1 out]
            n245 = disable-structure shown="RUN_TIME_ENGINE==False" {
              frame condition #0 (active) {
                # "functionality not available in exe"
                n246 = invoke on="Invoke Node" class="VI" method="Lock State.Get"() -> (error out=w306:errorcluster, "Get Lock State"=w305:T19, "pwd in cache"=w302:bool)  [unwired: 4 in, 1 out]
                n247 = Equal?(x=T19."Password-protected", y=w305) -> (x = y?=w303:bool)
                n248 = Compound Arithmetic op=AND(w303, invert w302) -> (w301:bool)
                n249 = case shown="False" w301 {
                  tunnel: w306 -> [w308 _]
                  frame False {
                    n250 = property on="Property Node" class="VI"(error in=w308, "BDWin.Open"=TRUE ("Block Diagram Window:Open")) -> ()  [unwired: 1 in, 2 out]
                  }
                  frame True {
                    # "Password-protected VI, and the password is not in the cache. Do not show the diagram."
                  }
                }
              }
              frame condition #1 {
              }
            }
          }
          event User Event {
            # "Show the panel of this VI, and send a status updated message to let listeners know."
            # "Another Module called the \"Show Panel\" API Method."
            n251 = event-data() -> ()  [unwired: 1 in, 1 out]
            n252 = control-ref of="This VI"() -> (w309:refnum<vi>)
            n253 = call "Open VI Panel.vi"("VI"=w309) -> ()  [unwired: 10 in, 1 out]
          }
          event User Event {
            # "The Stop Module Event can get fired from the Exit message in the MHL. The queue gets destroyed in that case. If the queue no longer exists, the Enqueue Exit as a priority message will return error 1. It is safe to ignore, because the module is already exiting."
            # "Another Module called the \"Stop Module\" API Method  or the Message Handling Loop below."
            n254 = event-data() -> ("Exit via Stop Module Req?"=w316:bool, "Wait for Module to stop?"=w315:bool)  [unwired: 1 in]
            n255 = Bundle By Name(cluster=T20 {"Origin"="", "Exit via Stop Module Req?"=FALSE, "Wait for Module to stop?"=FALSE} ("Stop Argument"), "Exit via Stop Module Req?"=w316, "Wait for Module to stop?"=w315) -> (w314:T20)
            n256 = call-poly <vilib>:"Delacor_lib_QMH_Enqueue Message (poly).vi"("Priority Message? (F)"=TRUE, "Message Data"=w314, "Message"="Exit", "Message Queue in"=w320) -> ("error out"=w324:errorcluster)  [unwired: 6 in, 1 out]
            n257 = call <vilib>:"Clear Errors.vi"("error in (no error)"=w324, "specific error code to clear (0: all)"=1) -> ("error out"=w323:errorcluster)  [unwired: 4 in, 1 out]
          }
          event Panel Close? {
            w330 = TRUE  # Discard the event, the MHL is responsible for closing and stopping this VI.
            # "Hide the panel or send the 'Exit' message if the user clicks the 'X' on the module main VI panel."
            n258 = event-data() -> ()  [unwired: 1 in, 1 out]
            n259 = call-poly <vilib>:"Delacor_lib_QMH_Enqueue Message (poly).vi"("Priority Message? (F)"=TRUE, "Message"="Exit", "Message Queue in"=w329) -> ("error out"=w331:errorcluster)  [unwired: 7 in, 1 out]
            n260 = event-data ("Event Filter Node")("Discard?"=w330) -> ()  [unwired: 1 in, 1 out]
          }
          event Timeout {
            w332 = FALSE  # Init?
            n261 = event-data() -> ()  [unwired: 1 in, 1 out]
            n262 = call "Scan For App Projects.vi"("Init?"=w332) -> ("error out"=w335:errorcluster)  [unwired: 10 in]
          }
          event User Event {
            # "Another Module called the \"Launch DQMH Scripting Tools\" API Method."
            n263 = event-data() -> ("Scripting Tool"=w336:T14)  [unwired: 1 in]
            n264 = Bundle(cluster=T13 {"Scripting Tool"=enum."Create New DQMH Event"} ("Launch DQMH Scripting Tools Argument"), "Scripting Tool"=w336) -> (w337:T13)
            n265 = call-poly <vilib>:"Delacor_lib_QMH_Enqueue Message (poly).vi"("Message Data"=w337, "Message"="Launch DQMH Scripting Tools", "Message Queue in"=w340) -> ("error out"=w343:errorcluster)  [unwired: 7 in, 1 out]
          }
          event User Event {
            # "Another Module called the \"Generate Project Documentation\" API Method."
            n266 = event-data() -> ("Boolean"=w344:bool)  [unwired: 1 in]
            n267 = Bundle(cluster=T21 {"Boolean"=FALSE} ("Generate Project Documentation Argument"), "Boolean"=w344) -> (w345:T21)
            n268 = call-poly <vilib>:"Delacor_lib_QMH_Enqueue Message (poly).vi"("Message Data"=w345, "Message"="Generate Project Documentation", "Message Queue in"=w348) -> ("error out"=w351:errorcluster)  [unwired: 7 in, 1 out]
          }
          event "Generate Antidoc": Value Change {
            # "Another Module called the \"Generate Project Documentation\" API Method."
            n269 = event-data() -> ()  [unwired: 1 in, 1 out]
            n270 = Bundle(cluster=T21 {"Boolean"=FALSE} ("Generate Project Documentation Argument"), "Boolean"="Generate Antidoc") -> (w353:T21)
            n271 = call-poly <vilib>:"Delacor_lib_QMH_Enqueue Message (poly).vi"("Message Data"=w353, "Message"="Generate Project Documentation", "Message Queue in"=w356) -> ("error out"=w359:errorcluster)  [unwired: 7 in, 1 out]
          }
          event User Event {
            # "Another Module called the \"Set App Theme\" API Method."
            n272 = event-data() -> ("Theme"=w360:bool)  [unwired: 1 in]
            n273 = Bundle(cluster=T22 {"Theme"=FALSE} ("Set App Theme Argument"), "Theme"=w360) -> (w361:T22)
            n274 = call-poly <vilib>:"Delacor_lib_QMH_Enqueue Message (poly).vi"("Message Data"=w361, "Message"="Set App Theme", "Message Queue in"=w364) -> ("error out"=w367:errorcluster)  [unwired: 7 in, 1 out]
          }
          event "Theme Panther": Value Change {
            # "Another Module called the \"Set App Theme\" API Method."
            n275 = event-data() -> ()  [unwired: 1 in, 1 out]
            n276 = Bundle(cluster=T22 {"Theme"=FALSE} ("Set App Theme Argument"), "Theme"="Theme Panther") -> (w369:T22)
            n277 = call-poly <vilib>:"Delacor_lib_QMH_Enqueue Message (poly).vi"("Message Data"=w369, "Message"="Set App Theme", "Message Queue in"=w372) -> ("error out"=w375:errorcluster)  [unwired: 7 in, 1 out]
          }
          event User Event {
            # "Another Module called the \"Show About\" API Method."
            n278 = event-data() -> ("Boolean"=w376:bool)  [unwired: 1 in]
            n279 = Bundle(cluster=T23 {"Boolean"=FALSE} ("Show About Argument"), "Boolean"=w376) -> (w377:T23)
            n280 = call-poly <vilib>:"Delacor_lib_QMH_Enqueue Message (poly).vi"("Message Data"=w377, "Message"="Show About", "Message Queue in"=w380) -> ("error out"=w383:errorcluster)  [unwired: 7 in, 1 out]
          }
          event "About Panther": Value Change {
            # "Another Module called the \"Show About\" API Method."
            n281 = event-data() -> ()  [unwired: 1 in, 1 out]
            n282 = Bundle(cluster=T23 {"Boolean"=FALSE} ("Show About Argument"), "Boolean"="About Panther") -> (w385:T23)
            n283 = call-poly <vilib>:"Delacor_lib_QMH_Enqueue Message (poly).vi"("Message Data"=w385, "Message"="Show About", "Message Queue in"=w388) -> ("error out"=w391:errorcluster)  [unwired: 7 in, 1 out]
          }
          event User Event {
            # "Another Module called the \"Update Module ID\" API Method."
            n284 = event-data() -> ("New ID"=w392:i32)  [unwired: 1 in]
            n285 = Bundle(cluster=T24 {"New ID"=-1} ("Update Module ID Argument"), "New ID"=w392) -> (w393:T24)
            n286 = call-poly <vilib>:"Delacor_lib_QMH_Enqueue Message (poly).vi"("Message Data"=w393, "Message"="Update Module ID", "Message Queue in"=w396) -> ("error out"=w399:errorcluster)  [unwired: 7 in, 1 out]
          }
          event "Module ID": Value Change {
            # "Another Module called the \"Update Module ID\" API Method."
            n287 = event-data() -> ()  [unwired: 1 in, 1 out]
            n288 = Bundle(cluster=T24 {"New ID"=-1} ("Update Module ID Argument"), "New ID"="Module ID") -> (w401:T24)
            n289 = call-poly <vilib>:"Delacor_lib_QMH_Enqueue Message (poly).vi"("Message Data"=w401, "Message"="Update Module ID", "Message Queue in"=w404) -> ("error out"=w407:errorcluster)  [unwired: 7 in, 1 out]
          }
          event User Event {
            # "Another Module called the \"Save Library Description\" API Method."
            n290 = event-data() -> ("Library Description"=w408:string)  [unwired: 1 in]
            n291 = Bundle(cluster=T25 {"Library Description"=""} ("Save Library Description Argument"), "Library Description"=w408) -> (w409:T25)
            n292 = call-poly <vilib>:"Delacor_lib_QMH_Enqueue Message (poly).vi"("Message Data"=w409, "Message"="Save Library Description", "Message Queue in"=w412) -> ("error out"=w415:errorcluster)  [unwired: 7 in, 1 out]
          }
          event User Event {
            # "Another Module called the \"Save VI Description\" API Method."
            n293 = event-data() -> ("VI Description"=w416:string)  [unwired: 1 in]
            n294 = Bundle(cluster=T26 {"VI Description"=""} ("Save VI Description Argument"), "VI Description"=w416) -> (w417:T26)
            n295 = call-poly <vilib>:"Delacor_lib_QMH_Enqueue Message (poly).vi"("Message Data"=w417, "Message"="Save VI Description", "Message Queue in"=w420) -> ("error out"=w423:errorcluster)  [unwired: 7 in, 1 out]
          }
          event User Event {
            # "Another Module called the \"Open Documentation\" API Method."
            n296 = event-data() -> ("Boolean"=w424:bool)  [unwired: 1 in]
            n297 = Bundle(cluster=T27 {"Boolean"=FALSE} ("Open Documentation Argument"), "Boolean"=w424) -> (w425:T27)
            n298 = call-poly <vilib>:"Delacor_lib_QMH_Enqueue Message (poly).vi"("Message Data"=w425, "Message"="Open Documentation", "Message Queue in"=w428) -> ("error out"=w431:errorcluster)  [unwired: 7 in, 1 out]
          }
          event "Open Antidoc Output": Value Change {
            # "Another Module called the \"Open Documentation\" API Method."
            n299 = event-data() -> ()  [unwired: 1 in, 1 out]
            n300 = Bundle(cluster=T27 {"Boolean"=FALSE} ("Open Documentation Argument"), "Boolean"="Open Antidoc Output") -> (w433:T27)
            n301 = call-poly <vilib>:"Delacor_lib_QMH_Enqueue Message (poly).vi"("Message Data"=w433, "Message"="Open Documentation", "Message Queue in"=w436) -> ("error out"=w439:errorcluster)  [unwired: 7 in, 1 out]
          }
          event User Event {
            # "Another Module called the \"Save Project Documentation\" API Method."
            n302 = event-data() -> ("Project Description"=w440:string)  [unwired: 1 in]
            n303 = Bundle(cluster=T28 {"Project Description"=""} ("Save Project Documentation Argument"), "Project Description"=w440) -> (w441:T28)
            n304 = call-poly <vilib>:"Delacor_lib_QMH_Enqueue Message (poly).vi"("Message Data"=w441, "Message"="Save Project Documentation", "Message Queue in"=w444) -> ("error out"=w447:errorcluster)  [unwired: 7 in, 1 out]
          }
        }
        n305 = call-dynamic "Delacor_lib_QMH_Error Handler - Event Handling Loop.vi"("error in"=w145, "Message Queue in"=w140) -> ("dup error in"=w144:errorcluster)  [unwired: 8 in, 1 out]
      }
      n306 = while {
        tunnel: w33 -> [w50]
        tunnel: [w49] -> w32
        shift-right: [w47] -> _
        shift-left: -1 -> [w46]
        shift-right: [w45] -> _
        shift-left: _ -> [w44]
        tunnel: w30 -> [w43]
        tunnel: [w51] -> w37
        shift-right: [w42] -> _
        shift-left: _ -> [w41]
        stop <- w48 stop-if-true
        # "Helper Loop"
        n307 = event shown="[3] <Panther Dashboard Broadcast Events.Projects Updated>: User Event" {
          selector: w50 -> [_ _ _ _ _ _ _ w112 _ _ _]
          dyn-events: [_ _ _ _ _ _ _ w110 _ _ _] -> w49
          timeout: w46 -> [_ _ _ _ _ _ _ _ _ _ _]
          tunnel: [_ TRUE _ _ _ _ _ _ _ _ _] -> w48
          tunnel: [w54 w59 w64 w77 w89 w93 w105 w111 w119 w130 w134] -> w45
          tunnel: [w55 w60 500 w76 w88 w92 w104 w114 w118 w129 w133] -> w47
          tunnel: w46 -> [w55 w60 _ w76 w88 w92 w104 w114 w118 w129 w133]
          tunnel: w44 -> [w54 w59 _ w77 w89 w93 w105 w111 w119 w130 w134]
          tunnel: [w56 _ _ _ _ _ _ _ w120 _ _] -> w52
          tunnel: [w53 w57 w62 w75 w86 w91 w103 w113 w117 w128 w132] -> w42
          tunnel: w41 -> [w53 w57 _ w75 w86 w91 w103 w113 w117 w128 w132]
          event Timeout {
            n308 = event-data() -> ()  [unwired: 1 in, 1 out]
            n309 = call "Get Module Execution Status by ref.vi"("Modules Tree ref"=w53, "Refs"=w54) -> ("error out"=w56:errorcluster)  [unwired: 9 in]
          }
          event User Event {
            n310 = event-data() -> ()  [unwired: 1 in, 1 out]
            n311 = Unbundle By Name(w59) -> ("Modules"=w58:refnum<vi>[])
            n312 = Close Reference(reference=w58) -> ()  [unwired: 1 in, 1 out]
          }
          event User Event {
            # "Refresh time"
            n313 = event-data() -> ("Modules"=w67:refnum<vi>[], "Modules Types"=w65:T9[], "Application Instance"=w66:refnum<vi>)  [unwired: 1 in]
            n314 = Bundle By Name(cluster=T11 {"Modules"=[], "Modules Types"=[], "Application Instance"=refnum}, "Modules"=w67, "Modules Types"=w65, "Application Instance"=w66) -> (w64:T11)
            n315 = control-ref of="Modules Tree"() -> (w63:refnum<vi>)
            n316 = call "Set Tree custom symbols.vi"("TreeControl in"=w63) -> ("TreeControl out"=w62:refnum<vi>)  [unwired: 10 in]
          }
          event User Event {
            n317 = event-data() -> ("Projects"=w73:string[])  [unwired: 1 in]
            n318 = Array Size(array=w73) -> (size(s)=w72:i32)
            n319 = Equal?(x=1, y=w72) -> (x = y?=w70:bool)
            n320 = control-ref of="Projects"() -> (w74:refnum<vi>)
            n321 = case shown="False" w70 {
              tunnel: w74 -> [w80 w83]
              tunnel: w73 -> [w79 w82]
              frame True {
                n322 = Index Array(array=w79) -> (element=w78:string)  [unwired: 1 in]
                n323 = property class="CmbBox"(reference=w80, "Strings[]"=w79, "Val(Sgnl)"=w78) -> ()  [unwired: 1 in, 2 out]
              }
              frame False {
                n324 = property class="CmbBox"(reference=w83, "Strings[]"=w82, "Text.Text"="") -> ()  [unwired: 1 in, 2 out]
              }
            }
          }
          event User Event {
            n325 = event-data() -> ("Targets"=w85:string[])  [unwired: 1 in]
            n326 = Index Array(array=w85) -> (element=w84:string)  [unwired: 1 in]
            n327 = control-ref of="Targets"() -> (w87:refnum<vi>)
            n328 = property class="CmbBox"(reference=w87, "Strings[]"=w85, "Value"=w84) -> ()  [unwired: 1 in, 2 out]
          }
          event User Event {
            n329 = event-data() -> ("Progress"=→"Progress":u16)  [unwired: 1 in]
          }
          event Mouse Enter {
            n330 = event-data() -> ("CtlRef"=w94:refnum<vi>)  [unwired: 1 in]
            n331 = property class="Ctl"(reference=w94) -> ("Label.Text"=w100:string, "TipStrip"=w101:string)  [unwired: 1 in, 2 out]
            n332 = control-ref of="antidoc"() -> (w95:refnum<vi>)
            n333 = control-ref of="Panther Indicator"() -> (w99:refnum<vi>)
            n334 = control-ref of="Process Indicator"() -> (w98:refnum<vi>)
            n335 = control-ref of="Event Indicator"() -> (w97:refnum<vi>)
            n336 = Empty String/Path?(string/path=w101) -> (empty?=w102:bool)
            n337 = Build Array(w95, w99, w98, w97) -> (w96:refnum<vi>[])
            n338 = call "Set Indicators Visibility Status.vi"("Indicator Refs"=w96, "Label"=w100) -> ()  [unwired: 10 in]
            n339 = case shown="False" w102 {
              tunnel: w101 -> [w106 _]
              frame False {
                n340 = call "Status Updated.vi"("Status"=w106) -> ()  [unwired: 10 in, 1 out]
              }
              frame True {
              }
            }
          }
          event User Event {
            n341 = event-data() -> ()  [unwired: 1 in, 1 out]
            n342 = control-ref of="This VI"() -> (w108:refnum<vi>)
            n343 = property class="VI"(reference=w108) -> ("Panel"=w109:refnum<vi>)  [unwired: 1 in, 2 out]
            n344 = property class="Pnl"(reference=w109) -> ("Controls[]"=w107:refnum<vi>[])  [unwired: 1 in, 2 out]
            n345 = register-events(reference=w112, w107) -> (reference out=w110:refnum<event-registration>)  [unwired: 3 in, 1 out]
          }
          event User Event {
            n346 = event-data() -> ("Scale Max"=w116:i32)  [unwired: 1 in]
            n347 = control-ref of="Progress"() -> (w115:refnum<vi>)
            n348 = property class="Slide (strict)"(reference=w115, "Scale.Maximum"=w116) -> (error out=w120:errorcluster)  [unwired: 1 in, 1 out]
          }
          event User Event {
            n349 = event-data() -> ("Module Type"=w127:T9)  [unwired: 1 in]
            n350 = Equal?(x=Module_type--enum."Module type: Cloneable", y=w127) -> (x = y?=w125:bool)
            n351 = Select(t=T12."Enabled" ("Disabled"), s=w125, f=T12."Disabled and Grayed Out") -> (s? t:f=w122:T12)
            n352 = control-ref of="Module ID"() -> (w124:refnum<vi>)
            n353 = property class="DigNum (strict)"(reference=w124, "DisabledEnum"=w122) -> ()  [unwired: 1 in, 2 out]
          }
          event User Event {
            n354 = event-data() -> ("Status"=→"Status":string)  [unwired: 1 in]
          }
        }
        n355 = call-dynamic "Delacor_lib_QMH_Error Handler - Helper Loop.vi"("error in"=w52, "Message Queue in"=w43) -> ("dup error in"=w51:errorcluster)  [unwired: 8 in, 1 out]
      }
    }
    frame Error {
      # "Synchronize Caller Events.vi will inform Start Module.vi that the module has launched and will let the code calling Start Module.vi register for broadcasts and would permit the caller receive the broadcast that an error occurred at launch time."
      n356 = call-dynamic "Delacor_lib_QMH_Release Message Queue.vi"("error in"=w805, "Message Queue"=w799) -> ("error out"=w804:errorcluster)  [unwired: 9 in]
      n357 = call "Synchronize Caller Events.vi"("Singleton Module Admin in"=w800) -> ("error out"=w806:errorcluster)  [unwired: 9 in, 1 out]
      n358 = call "Module Name--constant.vi"() -> ("Module Name"=w802:string)  [unwired: 11 in]
      n359 = Format Into String(format string="An error occurred during initialization. %s is no longer running.", w802) -> (resulting string=w797:string)  [unwired: 2 in, 1 out]
      n360 = Merge Errors(w804, w806) -> (w807:errorcluster)
      n361 = call "Stop Module.vi"("Origin"=w797) -> ()  [unwired: 10 in, 1 out]
      n362 = call "Error Reported.vi"("Additional Information"=w797, "Error"=w807) -> ()  [unwired: 9 in, 1 out]
    }
  }
  n363 = Merge Errors(w24, w26, w19) -> (w23:errorcluster)
  n364 = call "Close Module.vi"("error in (no error)"=w23, "Module Admin in"=w14) -> ("error out"=w25:errorcluster, "External Launch"=w8:bool, "Module Admin out"=w9:refnum<class "Delacor_lib_QMH_Module Admin.lvclass">)  [unwired: 7 in]
  n365 = Unregister For Events(event registration refnum=w6) -> ()  [unwired: 1 in, 1 out]
  n366 = Unregister For Events(event registration refnum=w13, error in=w25) -> (error out=w22:errorcluster)
  "error out" <- w22
  n367 = case "External Launch?" shown="True" w8 {
    tunnel: w22 -> [_ w808]
    frame False {
    }
    frame True {
      n368 = case shown="No Error" w808 {
        frame No Error {
          n369 = invoke class="VI" method="FP.Close"() -> ()  [unwired: 3 in, 3 out]
        }
        frame Error {
          n370 = invoke on="Invoke Node" class="VI" method="FP.Open"("Activate"=TRUE ("Activate?")) -> ()  [unwired: 4 in, 5 out]
        }
      }
    }
  }
  n371 = local write "Module Admin"(w9) -> ()
